vi "Init.vi"(8 "error in (no error)":errorcluster, 10 "ID":string, 11 "Mixer in":refnum<class "Mixer.lvclass">) -> (0 "error out":errorcluster, 3 "Mixer out":refnum<class "Mixer.lvclass">)   [LabVIEW 2018, in "Mixer.lvclass"]
uses:
  Mixer.lvclass
  Libraries/Audio Processing/Value Cluster.ctl
  Libraries/Audio Processing/Value Properties.ctl
  Mixer.lvclass/Mixer.ctl
  Channel/Channel.lvclass
  Libraries/Messaging/Messaging.lvlib
  Libraries/Audio Processing/Audio Processing.lvlib
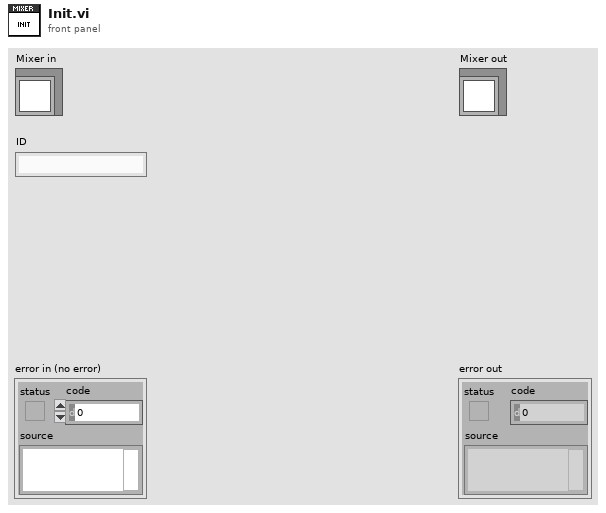
[diagram p1: front panel]
types:
  T1 = typedef "Audio Processing.lvlib/Value Cluster.ctl" = cluster{"Value":dbl, "Limits":T2}
  T2 = typedef "Audio Processing.lvlib/Value Properties.ctl" = cluster{"Lower":dbl, "Upper":dbl}
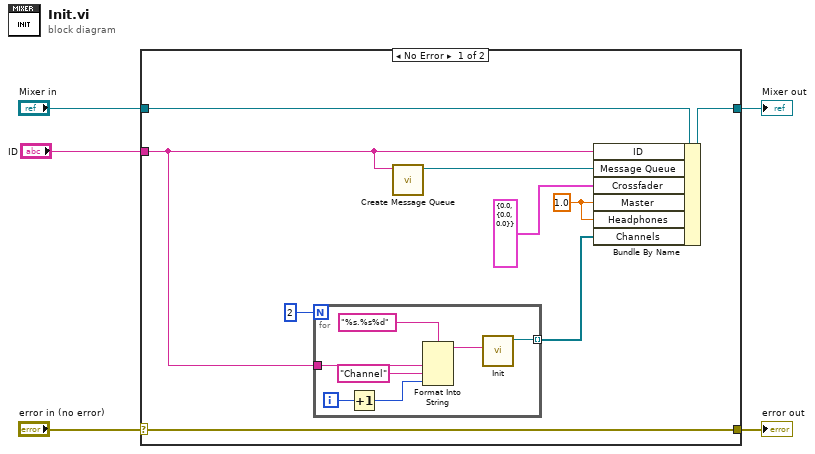
[diagram p0: block diagram]
diagram:
  n1 = case shown="No Error" "error in (no error)" {
    selector: "error in (no error)" -> [w14 w23]
    tunnel: [w14 w23] -> w4
    tunnel: [w13 w22] -> w2
    tunnel: "Mixer in" -> [w12 w22]
    tunnel: "ID" -> [w8 _]
    frame No Error {
      w9 = 1.0 ("Master Volume")
      n2 = for {
        N: 2 -> [_]
        tunnel: w8 -> [w21]
        tunnel: [w15] -> w11 mode=indexing
        i -> [w19]
        n3 = Increment(x=w19) -> (x+1=w18:i32)
        n4 = Format Into String(format string="%s.%s%d", w21, "Channel" ("input 2"), w18) -> (resulting string=w16:string)  [unwired: 2 in, 1 out]
        n5 = call "Init.vi"("ID"=w16) -> ("Channel out"=w15:refnum<class "Channel.lvclass">)  [unwired: 9 in, 1 out]
      }
      n6 = call "Create Message Queue.vi"("Queue Name"=w8) -> ("queue out"=w7:refnum<queue>)  [unwired: 9 in, 1 out]
      n7 = Bundle By Name(cluster=w12, "ID"=w8, "Message Queue"=w7, "Crossfader"=T1 {"Value"=0.0, "Limits"={"Lower"=0.0, "Upper"=0.0}}, "Master"=w9, "Headphones"=w9, "Channels"=w11) -> (w13:refnum<class "Mixer.lvclass">)
    }
    frame Error {
    }
  }
  "error out" <- w4
  "Mixer out" <- w2
